vi "Valid Plugin Name.vi"(8 "error in":errorcluster, 10 "requested plugin name":string, 11 "project ref":refnum<vi>) -> (0 "error out":errorcluster, 3 "valid name?":bool)   [LabVIEW 2021, in "InstrumentStudio Plug-In Editor.lvlib"]
uses:
  InstrumentStudio Plug-In Editor.lvlib
  48953c88-0603-4c13-ba6a-df914321b09e.vi
  <vilib>/Comparison/Equal/Equal Functor/Equal Functor.lvclass
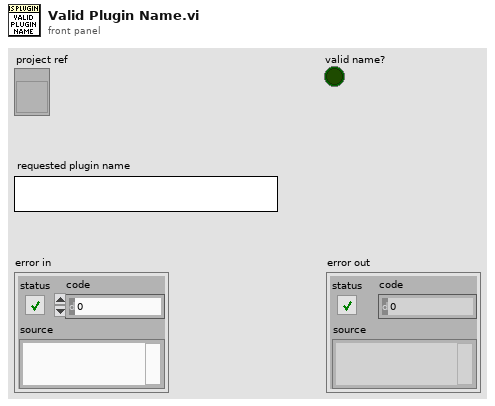
[diagram p1: front panel]
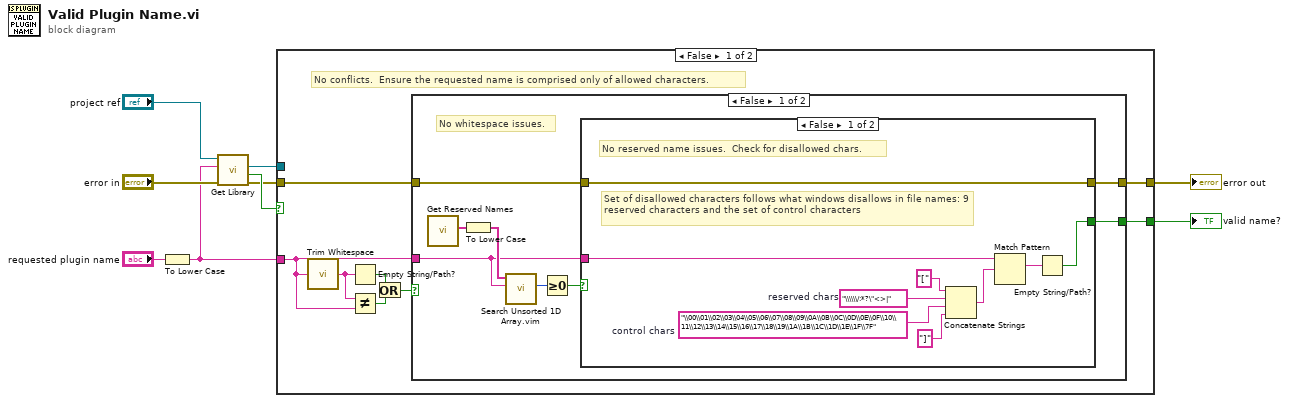
[diagram p0: block diagram]
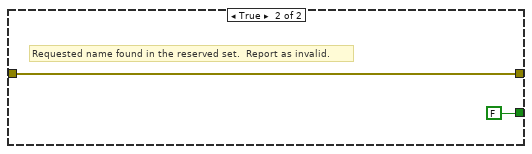
[diagram p2: hidden frame]
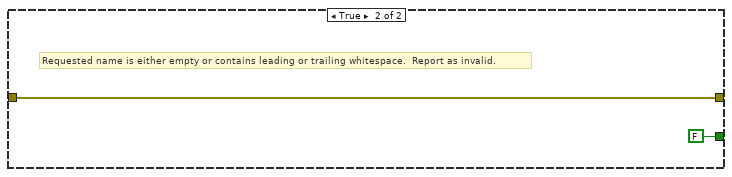
[diagram p3: hidden frame]
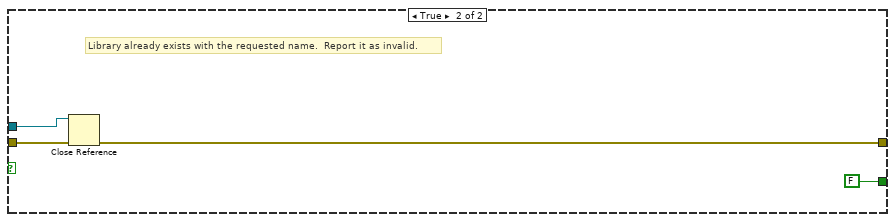
[diagram p4: hidden frame]
diagram:
  n1 = To Lower Case(string="requested plugin name") -> (all lower case string=w1:string)
  n2 = call "Get Library.vi"("error in"="error in", "library name"=w1, "project ref"="project ref") -> ("error out"=w6:errorcluster, "found"=w7:bool, "library item"=w5:refnum<vi>)  [unwired: 5 in, 1 out]
  n3 = case shown="False" w7 {
    tunnel: w6 -> [w17 w42]
    tunnel: w5 -> [_ w40]
    tunnel: [w16 w41] -> w4
    tunnel: [w15 FALSE ("Valid Name?")] -> w3
    tunnel: w1 -> [w10 _]
    frame False {
      # "No conflicts.  Ensure the requested name is comprised only of allowed characters."
      n4 = call <vilib>:"Trim Whitespace.vi"("string"=w10) -> ("trimmed string"=w14:string)  [unwired: 1 in]
      n5 = Empty String/Path?(string/path=w14) -> (empty?=w12:bool)
      n6 = Not Equal?(x=w14, y=w10) -> (x != y?=w13:bool)
      n7 = Or(x=w12, y=w13) -> (x .or. y?=w11:bool)
      n8 = case shown="False" w11 {
        tunnel: w10 -> [w21 _]
        tunnel: w17 -> [w25 w38]
        tunnel: [w24 w38] -> w16
        tunnel: [w18 FALSE ("Error if not Found (T)")] -> w15
        frame False {
          # "No whitespace issues."
          n9 = call "Get Reserved Names.vi"() -> ("reserved names"=w23:string[])  [unwired: 11 in]
          n10 = To Lower Case(string=w23) -> (all lower case string=w22:string[])
          n11 = call "Search Unsorted 1D Array.vim"("element"=w21, "unsorted 1D array"=w22) -> ("index of element"=w20:i32)  [unwired: 9 in]
          n12 = Greater Or Equal To 0?(x=w20) -> (x >= 0?=w19:bool)
          n13 = case shown="False" w19 {
            tunnel: w21 -> [w33 _]
            tunnel: w25 -> [w34 w36]
            tunnel: [w34 w36] -> w24
            tunnel: [w31 FALSE ("Error if not Found (T)")] -> w18
            frame False {
              w26 = "\\00\\01\\02\\03\\04\\05\\06\\07\\08\\09\\0A\\0B\\0C\\0D\\0E\\0F\\10\\11\\12\\13\\14\\15\\16\\17\\18\\19\\1A\\1B\\1C\\1D\\1E\\1F\\7F"  # control chars
              w30 = "\\\\\\/:*?\"<>|"  # reserved chars
              # "Set of disallowed characters follows what windows disallows in file names: 9 reserved characters and the set of control characters"
              # "No reserved name issues.  Check for disallowed chars."
              n14 = Concatenate Strings("[" ("string"), w30, w26, "]" ("string")) -> (w27:string)
              n15 = Match Pattern(string=w33, regular expression=w27) -> (match substring=w32:string)  [unwired: 1 in, 3 out]
              n16 = Empty String/Path?(string/path=w32) -> (empty?=w31:bool)
            }
            frame True {
              # "Requested name found in the reserved set.  Report as invalid."
            }
          }
        }
        frame True {
          # "Requested name is either empty or contains leading or trailing whitespace.  Report as invalid."
        }
      }
    }
    frame True {
      # "Library already exists with the requested name.  Report it as invalid."
      n17 = Close Reference(reference=w40, error in (no error)=w42) -> (error out=w41:errorcluster)
    }
  }
  "error out" <- w4
  "valid name?" <- w3
